vi "Dilation.vi"() -> ()   [LabVIEW 2018]
doc: "Dilation: This example is an example of image dilation processing. This example is mainly used to enhance the boundaries of objects in images or fill voids in images, in order to better identify targets or perform subsequent analysis. In the dilation operation, each pixel in the image is considered as an element of a set, which is composed of the neighborhoods around the pixels. For each pixel, the dilation operation sets its value to the maximum value in the neighborhood."
uses:
  vi.lib/VIRobotics/opencv_yiku/Mat/Mat_8U/Mat_8U.lvclass
  C:/Program Files/National Instruments/LabVIEW 2018/vi.lib/VIRobotics/opencv_yiku/Mat/Mat/Mat.lvclass
  vi.lib/VIRobotics/opencv_yiku/Mat/Create_Mat_8U.vi
  vi.lib/VIRobotics/opencv_yiku/opencv_yiku.lvlib
panel:
  out "picture":picture
  in  "shape":T1(ring)
  in  "size":cluster{"x":i32, "y":i32}={"x"=3, "y"=3}
  out "dilate picture":picture
  # "Overview: Here, a pixel element is '1' if at least one pixel under the kernel is '1'. So it increases the white region in the image or size of foreground object increases. Normally, in cases like noise removal, erosion is followed by dilation. Because, erosion removes white noises, but it also shrinks our object. So we dilate it. Since noise is gone, they won't come back, but our object area increases. It is also useful in joining broken parts of an object.\nRequirements: Windows.\nInstructions: \n1.Run the VI"
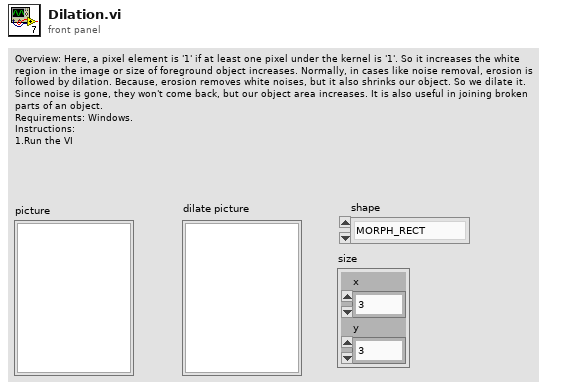
[diagram p1: front panel]
types:
  T1 = enum16{"MORPH_RECT", "MORPH_CROSS", "MORPH_ELLIPSE"}
  T2 = enum32{"COLOR_BGR2BGRA", "COLOR_BGRA2BGR", "COLOR_BGR2RGBA", "COLOR_RGBA2BGR", "COLOR_BGR2RGB", "COLOR_BGRA2RGBA", "COLOR_BGR2GRAY", "COLOR_RGB2GRAY", "COLOR_GRAY2BGR", "COLOR_GRAY2BGRA"}
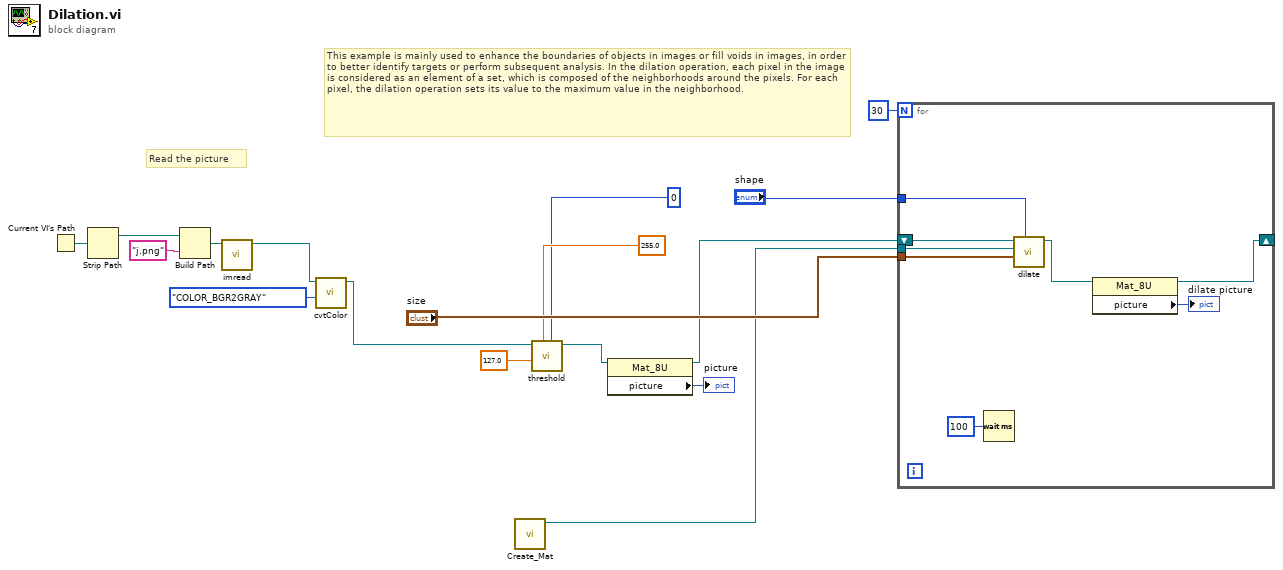
[diagram p0: block diagram]
diagram:
  # "This example is mainly used to enhance the boundaries of objects in images or fill voids in images, in order to better identify targets or perform subsequent analysis. In the dilation operation, each pixel in the image is considered as an element of a set, which is composed of the neighborhoods around the pixels. For each pixel, the dilation operation sets its value to the maximum value in the neighborhood."
  # "Read the picture"
  n1 = Current VI's Path() -> (path=w16:path)
  n2 = Strip Path(path=w16) -> (stripped path=w17:path)  [unwired: 1 out]
  n3 = Build Path(base path=w17, name or relative path="j.png") -> (appended path=w14:path)
  n4 = call "imread.vi"("path"=w14) -> ("Mat out"=w11:refnum<class "Mat_8U.lvclass">)  [unwired: 9 in, 1 out]
  n5 = call "cvtColor.vi"("dstCn"=T2."COLOR_BGR2GRAY", "src"=w11) -> ("src out"=w6:refnum<class "Mat_8U.lvclass">)  [unwired: 7 in, 2 out]
  n6 = call-poly "Create_Mat.vi"() -> ("Mat_8U_out"=w2:refnum<class "Mat_8U.lvclass">)  [unwired: 10 in, 1 out]
  n7 = call "threshold.vi"("type"=0, "maxval"=255.0, "thresh"=127.0, "Mat in"=w6) -> ("dst out"=w4:refnum<class "Mat_8U.lvclass">)  [unwired: 6 in, 1 out]
  n8 = property class="Mat_8U"(reference=w4) -> (reference out=w3:refnum<class "Mat_8U.lvclass">, "picture"=→"picture":picture)  [unwired: 1 in, 1 out]
  n9 = for {
    N: 30 -> [_]
    tunnel: "size" -> [w25]
    tunnel: "shape" -> [w24]
    tunnel: w2 -> [w22]
    shift-right: [w19] -> _
    shift-left: w3 -> [w23]
    n10 = Wait (ms)(milliseconds to wait=u32 100) -> ()  [unwired: 1 out]
    n11 = call "dilate.vi"("shape"=w24, "size"=w25, "dst in"=w22, "Mat in"=w23) -> ("dst out"=w20:refnum<class "Mat_8U.lvclass">)  [unwired: 6 in, 1 out]
    n12 = property class="Mat_8U"(reference=w20) -> (reference out=w19:refnum<class "Mat_8U.lvclass">, "picture"=→"dilate picture":picture)  [unwired: 1 in, 1 out]
  }
